vi "EditOptions.vi"(8 "error in":errorcluster, 11 "node in":refnum<class "VI modification collection.lvclass">) -> (0 "error out":errorcluster, 1 "edit options":T1, 2 "subnodes class":T2, 3 "node out":refnum<class "VI modification collection.lvclass">)   [LabVIEW 2013, in "VI modification collection.lvclass"]
doc: "Contains the options for the Menu that will be displayed when doing right click on an item.\nThe sub nodes class configures which nodes can be added to this nodes\nAnd the edit options determine which options are available for the node.\nThis configuration is stored in this VI in case some dynamic configuration is required for the menu options or sub nodes."
uses:
  VI modification collection.lvclass
  <vilib>/NI/Configuration Framework/Node/SubNodeCluster.ctl
  <vilib>/NI/Configuration Framework/Node/NodeMenuOptions.ctl
  VI modification.lvclass
  available modifications.vi
  <vilib>/NI/Configuration Framework/Node/NISE_CEF_Node.lvclass
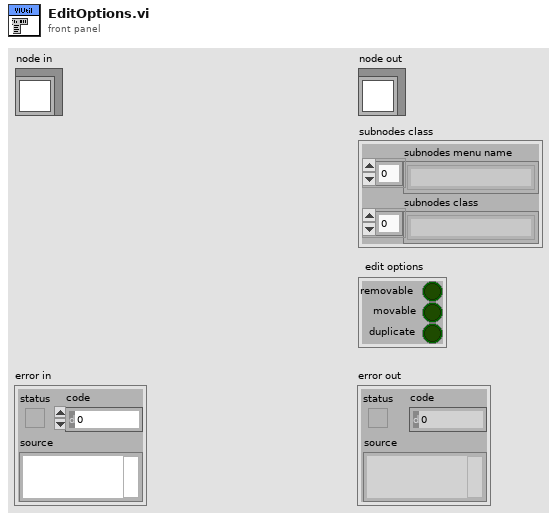
[diagram p1: front panel]
types:
  T1 = typedef "NISE_CEF_Node.lvclass/NodeMenuOptions.ctl" = cluster{"removable":bool, "movable":bool, "duplicate":bool}
  T2 = typedef "NISE_CEF_Node.lvclass/SubNodeCluster.ctl" = cluster{"subnodes menu name":string[], "subnodes class":string[]}
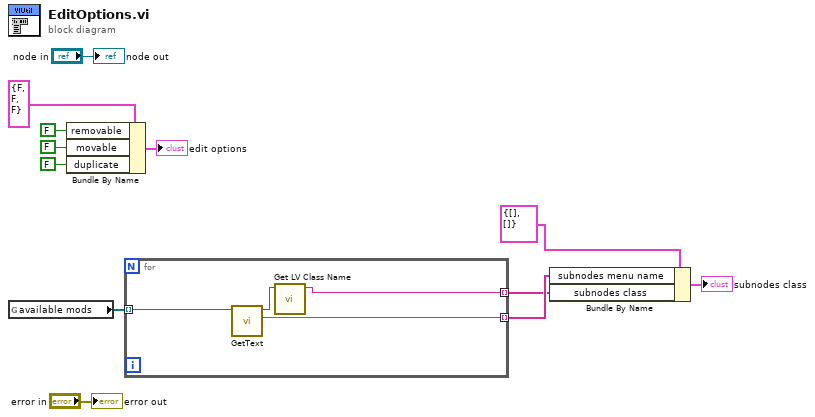
[diagram p0: block diagram]
diagram:
  n1 = global read "available modifications.vi" "available mods"() -> (w3:refnum<class "VI modification.lvclass">[])
  n2 = Bundle By Name(cluster=T1 {"removable"=FALSE, "movable"=FALSE, "duplicate"=FALSE} ("edit options"), "removable"=FALSE ("Removable"), "movable"=FALSE ("Movable"), "duplicate"=FALSE) -> (→"edit options":T1)
  n3 = for {
    tunnel: w3 -> [w16] mode=indexing
    tunnel: [w14] -> w2 mode=indexing
    tunnel: [w13] -> w1 mode=indexing
    n4 = call-dynamic "GetText.vi"("node in"=w16) -> ("text"=w14:string, "node out"=w15:refnum<class "VI modification.lvclass">)  [unwired: 6 in, 3 out]
    n5 = call <vilib>:"Get LV Class Name.vi"("object"=w15) -> ("class name"=w13:string)  [unwired: 9 in, 1 out]
  }
  n6 = Bundle By Name(cluster=T2 {"subnodes menu name"=[], "subnodes class"=[]} ("subnodes class"), "subnodes menu name"=w2, "subnodes class"=w1) -> (→"subnodes class":T2)
  "error out" <- "error in"
  "node out" <- "node in"
